vi "温度 1.vi"() -> ()   [LabVIEW 2014]
panel:
  out "温度值":dbl
  in  "温度值单位":bool
  out "温度计":dbl(slide) scale=0.0..100.0
  in  "采集的电压":dbl
  # "摄氏"
  # "华氏"
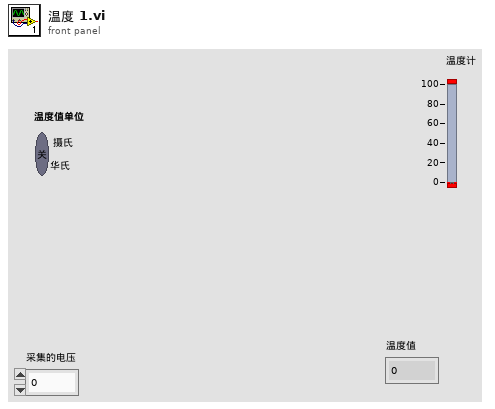
[diagram p1: front panel]
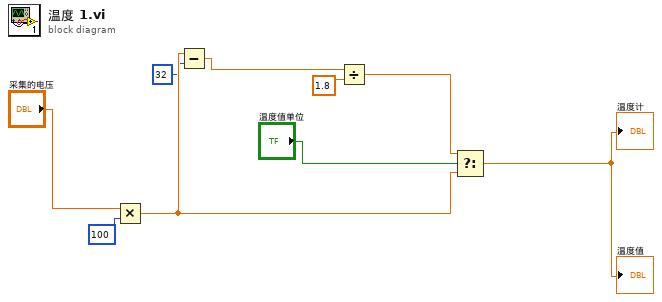
[diagram p0: block diagram]
diagram:
  n1 = Multiply(x="采集的电压", y=100) -> (x*y=w5:dbl)
  n2 = Subtract(x=w5, y=32) -> (x-y=w3:dbl)
  n3 = Divide(x=w3, y=1.8) -> (x/y=w1:dbl)
  n4 = Select(t=w1, s="温度值单位", f=w5) -> (s? t:f=→"温度计" →"温度值":dbl)
